vi "pH calibration.vi"(11 "pH index":i32) -> ()   [LabVIEW 2012]
uses:
  DAQ configuration/scale type.ctl
  DAQ configuration/Sensor buffer command.ctl
  global scale array.vi
panel:
  in  "Default Buffers":T1(array[cluster])=[{"Buffer"=4.0, "Calibrated"=FALSE, "V/T"=0.0013599919516459151}, {"Buffer"=7.0, "Calibrated"=FALSE, "V/T"=0.0}, {"Buffer"=10.0, "Calibrated"=FALSE, "V/T"=0.0}] {"V/T" format="%.2f"; "Buffer" format="%.2f"}
  out "name":string
  out "units":string
  in  "Temperature\nChannel":i32 min=0 step=1
  in  "Temperature":dbl[unit]=273.15 format="%.1f"
  in  "Temperature\ncompensated":bool
  out "XY Graph":cluster{dbl[], dbl[]}[](graph)
  in  "OK Button":bool
  in  "add buffer smooth interval (s)":sgl=1.0 format="%.3f"
  in  "Clear buffers":bool
  in  "Edit buffers":bool
  in  "Add buffer":bool
  out "Quit":bool
  out "Buffers":T1(array[cluster]) {"V/T" format="%.2f"; "Buffer" format="%.2f"}
  out "Sample Temperature":dbl[unit] format="%.2f"
  out "pH":dbl format="%.3f"
  out "pH voltage":sgl[unit] format="%.1f"
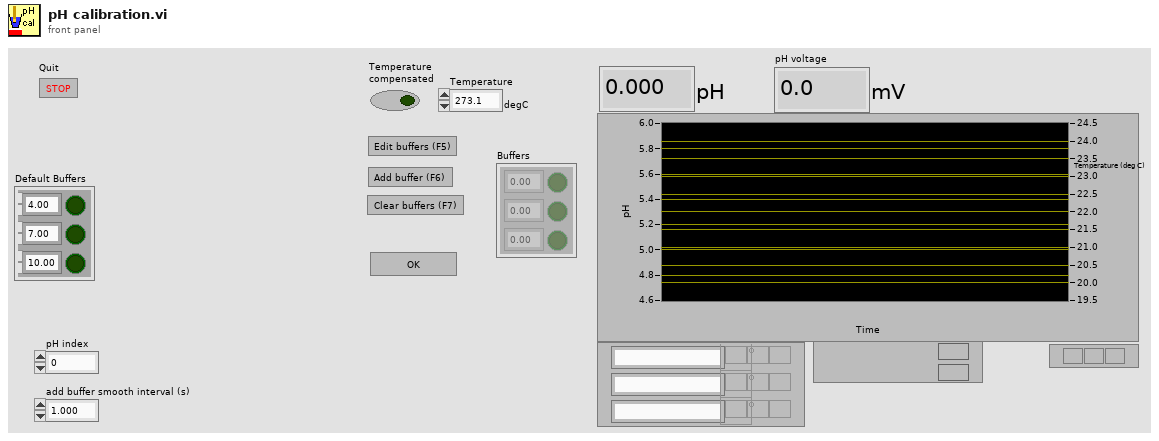
[diagram p1: front panel]
types:
  T1 = cluster{"Buffer":dbl, "Calibrated":bool, "V/T":dbl}[]
  T2 = typedef "scale type.ctl" = enum16{"Volts", "Polynomial", "Correspondence Table", "pH", "Dissolved Oxygen", "Quadratic"}
  T3 = typedef "Sensor buffer command.ctl" = enum16{"read average", "read recent", "read all", "write", "configure", "clear"}
  T4 = typedef "calib array.ctl" = T5[]
  T5 = typedef "conversion.ctl" = cluster{"conversion matrix":sgl[][], "units":string, "name":string, "scale type":T2, "offset (volts)":dbl, "second channel":i8, "correspondence table":T6, "offset (physical units)":dbl, "pH scale":T7, "D.O.":T8}
  T6 = typedef "correspondence table.ctl" = cluster{"physical units":dbl, "volts":dbl}[]
  T7 = typedef "pH scale.ctl" = cluster{"Buffers":cluster{"Buffer":dbl, "Calibrated":bool, "V/T":dbl}[], "Temperature":dbl}
  T8 = typedef "DO scale.ctl" = cluster{"Temperature":dbl, "K":dbl, "barometric pressure":dbl}
  T9 = cluster{"Buffer":dbl, "Calibrated":bool, "V/T":dbl}
  T10 = typedef "Sensor data.ctl" = cluster{" Sensor array":T11[], "Time":dbl}
  T11 = typedef "sensor cluster.ctl" = cluster{"voltage":sgl, "scaled":sgl, "units":string, "Out of Range":bool}
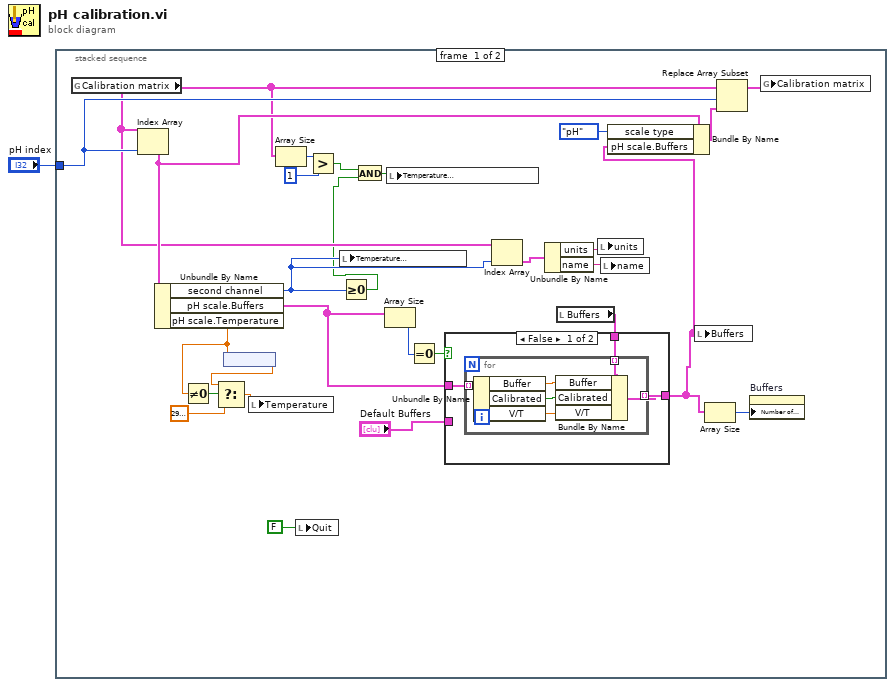
[diagram p0: block diagram]
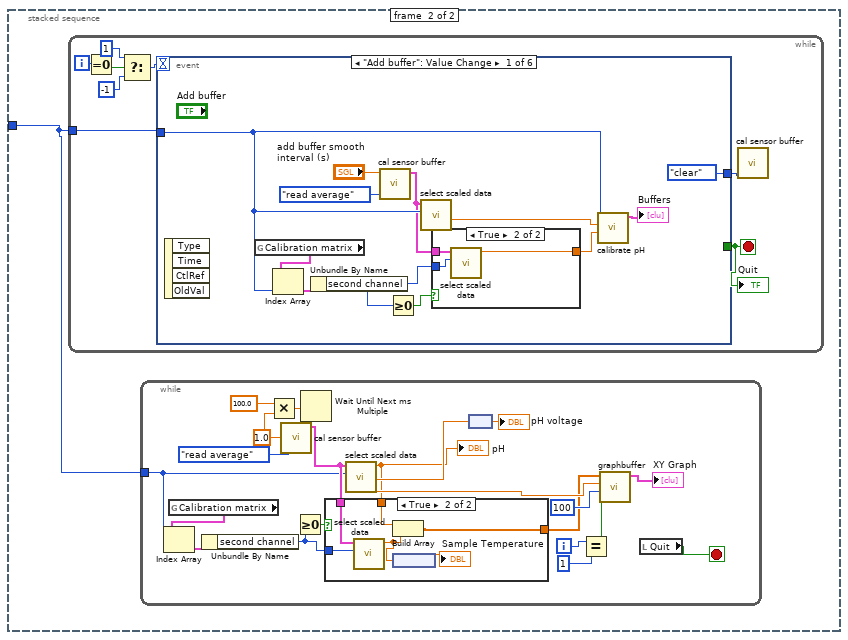
[diagram p3: hidden frame]
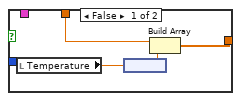
[diagram p4: hidden frame]
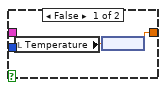
[diagram p5: hidden frame]
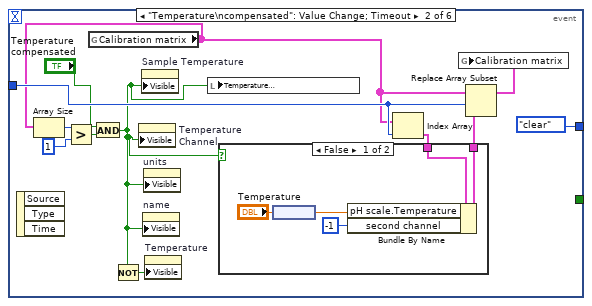
[diagram p6: hidden frame]
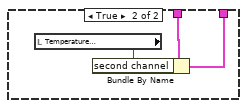
[diagram p7: hidden frame]
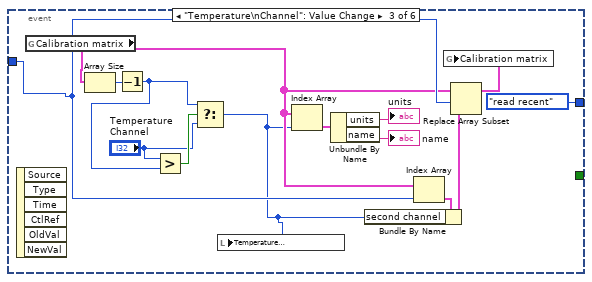
[diagram p8: hidden frame]
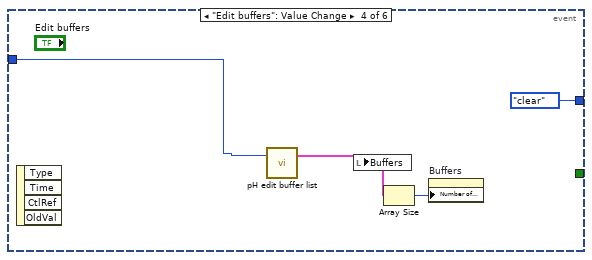
[diagram p9: hidden frame]
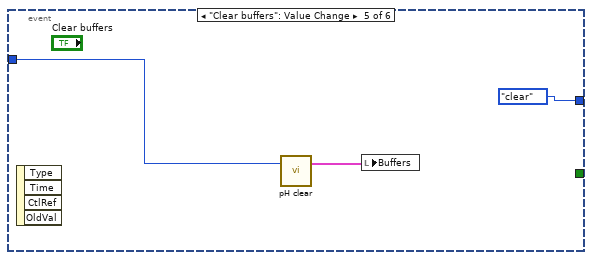
[diagram p10: hidden frame]
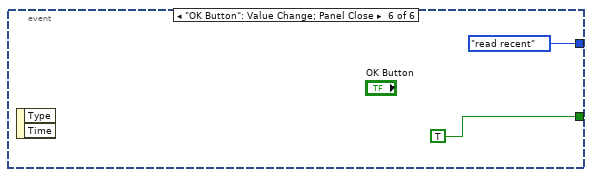
[diagram p11: hidden frame]
diagram:
  n1 = stacked-sequence {
    tunnel: "pH index" -> [w19 w40]
    frame #0 {
      n2 = global read "global scale array.vi" "Calibration matrix"() -> (w11:T4)
      n3 = Index Array(array=w11, index=w19) -> (element=w17:T5)
      n4 = Unbundle By Name(w17) -> ("second channel"=w27:i8, "pH scale.Buffers"=w23:T1, "pH scale.Temperature"=w7:dbl)
      n5 = Not Equal To 0?(x=w7) -> (x != 0?=w6:bool)
      n6 = node(w7) -> (w5:dbl[unit])
      n7 = Select(t=w5, s=w6, f=dbl[unit] 295.15) -> (s? t:f=w4:dbl[unit])
      n8 = local write "Temperature"(w4) -> ()
      n9 = Array Size(array=w11) -> (size(s)=w13:i32)
      n10 = local write "Quit"(FALSE ("Quit")) -> ()
      n11 = Greater?(x=w13, y=1) -> (0:w10:bool)
      n12 = local write "Temperature\nChannel"(w27) -> ()
      n13 = Greater Or Equal To 0?(x=w27) -> (x >= 0?=w9:bool)
      n14 = And(x=w10, y=w9) -> (x .and. y?=w8:bool)
      n15 = Array Size(array=w23) -> (size(s)=w21:i32)
      n16 = local write "Temperature\ncompensated"(w8) -> ()
      n17 = Equal To 0?(x=w21) -> (x = 0?=w22:bool)
      n18 = Index Array(array=w11, index=w27) -> (element=w26:T5)
      n19 = Unbundle By Name(w26) -> ("units"=w25:string, "name"=w24:string)
      n20 = local read "Buffers"() -> (w28:T1)
      n21 = case shown="False" w22 {
        tunnel: w23 -> [w32 _]
        tunnel: w28 -> [w31 _]
        tunnel: [w30 w39] -> w14
        tunnel: "Default Buffers" -> [_ w39]
        frame False {
          n22 = for {
            tunnel: w32 -> [w38] mode=indexing
            tunnel: w31 -> [w37] mode=indexing
            tunnel: [w34] -> w30 mode=indexing
            n23 = Unbundle By Name(w38) -> ("Buffer"=w36:dbl, "Calibrated"=w35:bool, "V/T"=w33:dbl)
            n24 = Bundle By Name(cluster=w37, "Buffer"=w36, "Calibrated"=w35, "V/T"=w33) -> (w34:T9)
          }
        }
        frame True {
        }
      }
      n25 = local write "units"(w25) -> ()
      n26 = local write "name"(w24) -> ()
      n27 = Bundle By Name(cluster=w17, "scale type"=scale_type."pH", "pH scale.Buffers"=w14) -> (w16:T5)
      n28 = local write "Buffers"(w14) -> ()
      n29 = Array Size(array=w14) -> (size(s)=w29:i32)
      n30 = Replace Array Subset(array=w11, new element=w16, index=w19) -> (w18:T4)
      n31 = property on="Buffers" class="Arr (strict)"("Number of Rows"=w29) -> ()  [unwired: 2 in, 2 out]
      n32 = global write "global scale array.vi" "Calibration matrix"(w18) -> ()
    }
    frame #1 {
      n33 = while {
        tunnel: w40 -> [w78]
        i -> [w74]
        stop <- w79 stop-if-true
        n34 = Equal To 0?(x=w74) -> (x = 0?=w73:bool)
        n35 = Select(t=1, s=w73, f=-1) -> (s? t:f=w75:i32)
        n36 = event shown="[0] \"Add buffer\": Value Change" {
          selector: _ -> [_ _ _ _ _ _]
          dyn-events: _ -> [_ _ _ _ _ _]
          timeout: w75 -> [_ _ _ _ _ _]
          tunnel: [_ _ _ _ _ TRUE ("OK Button")] -> w79
          tunnel: w78 -> [w91 w104 w126 w132 w136 _]
          tunnel: [Sensor_buffer_command."clear" ("command") Sensor_buffer_command."clear" ("command") Sensor_buffer_command."read recent" ("command") Sensor_buffer_command."clear" ("command") Sensor_buffer_command."clear" ("command") Sensor_buffer_command."read recent" ("command")] -> w72
          event "Add buffer": Value Change {
            n37 = event-data() -> ()  [unwired: 1 in, 4 out]
            n38 = global read "global scale array.vi" "Calibration matrix"() -> (w83:T4)
            n39 = Index Array(array=w83, index=w91) -> (element=w84:T5)
            n40 = Unbundle By Name(w84) -> ("second channel"=w82:i8)
            n41 = call "cal sensor buffer.vi"("command"=Sensor_buffer_command."read average", "smooth interval (s)"="add buffer smooth interval (s)") -> ("Sensor Data smoothed"=w88:T10)  [unwired: 3 in, 2 out]
            n42 = Greater Or Equal To 0?(x=w82) -> (x >= 0?=w81:bool)
            n43 = call "select scaled data.vi"("Sensor index"=w91, "Sensor Data"=w88) -> ("voltage"=w89:sgl)  [unwired: 4 in, 5 out]
            n44 = case shown="True" w81 {
              tunnel: w88 -> [_ w96]
              tunnel: [w92 w95] -> w86
              tunnel: w82 -> [_ w94]
              frame False {
                n45 = local read "Temperature"() -> (w93:dbl[unit])
                n46 = node(w93) -> (w92:dbl)
              }
              frame True {
                n47 = call "select scaled data.vi"("Sensor index"=w94, "Sensor Data"=w96) -> ("scaled"=w95:sgl)  [unwired: 4 in, 5 out]
              }
            }
            n48 = call "calibrate pH.vi"("index"=w91, "pH voltage"=w89, "Temperature"=w86) -> ("Buffers"=→"Buffers":T1)  [unwired: 7 in]
          }
          event "Temperature\ncompensated": Value Change; Timeout {
            n49 = event-data() -> ()  [unwired: 1 in, 3 out]
            n50 = global read "global scale array.vi" "Calibration matrix"() -> (w102:T4)
            n51 = Array Size(array=w102) -> (size(s)=w101:i32)
            n52 = Greater?(x=w101, y=1) -> (0:w99:bool)
            n53 = And(x="Temperature\ncompensated", y=w99) -> (x .and. y?=w97:bool)
            n54 = Not(x=w97) -> (.not. x?=w108:bool)
            n55 = property on="Temperature\nChannel" class="DigNum (strict)"("Visible"=w97) -> ()  [unwired: 2 in, 2 out]
            n56 = property on="Sample Temperature" class="DigNum (strict)"("Visible"=w97) -> ()  [unwired: 2 in, 2 out]
            n57 = property on="name" class="Str"("Visible"=w97) -> ()  [unwired: 2 in, 2 out]
            n58 = property on="units" class="Str"("Visible"=w97) -> ()  [unwired: 2 in, 2 out]
            n59 = property on="Temperature" class="DigNum (strict)"("Visible"=w108) -> ()  [unwired: 2 in, 2 out]
            n60 = local write "Temperature\ncompensated"(w97) -> ()
            n61 = Index Array(array=w102, index=w104) -> (element=w106:T5)
            n62 = case shown="False" w97 {
              tunnel: w106 -> [w113 w115]
              tunnel: [w112 w114] -> w105
              frame False {
                n63 = node("Temperature") -> (w110:dbl)
                n64 = Bundle By Name(cluster=w113, "pH scale.Temperature"=w110, "second channel"=i8 -1) -> (w112:T5)
              }
              frame True {
                n65 = local read "Temperature\nChannel"() -> (w116:i32)
                n66 = Bundle By Name(cluster=w115, "second channel"=w116) -> (w114:T5)
              }
            }
            n67 = Replace Array Subset(array=w102, new element=w105, index=w104) -> (w107:T4)
            n68 = global write "global scale array.vi" "Calibration matrix"(w107) -> ()
          }
          event "Temperature\nChannel": Value Change {
            n69 = event-data() -> ()  [unwired: 1 in, 6 out]
            n70 = global read "global scale array.vi" "Calibration matrix"() -> (w123:T4)
            n71 = Array Size(array=w123) -> (size(s)=w122:i32)
            n72 = Decrement(x=w122) -> (x-1=w120:i32)
            n73 = Greater?(x="Temperature\nChannel", y=w120) -> (0:w121:bool)
            n74 = Select(t=w120, s=w121, f="Temperature\nChannel") -> (s? t:f=w118:i32)
            n75 = local write "Temperature\nChannel"(w118) -> ()
            n76 = Index Array(array=w123, index=w118) -> (element=w130:T5)
            n77 = Unbundle By Name(w130) -> ("units"=→"units":string, "name"=→"name":string)
            n78 = Index Array(array=w123, index=w126) -> (element=w124:T5)
            n79 = Bundle By Name(cluster=w124, "second channel"=w118) -> (w125:T5)
            n80 = Replace Array Subset(array=w123, new element=w125, index=w126) -> (w127:T4)
            n81 = global write "global scale array.vi" "Calibration matrix"(w127) -> ()
          }
          event "Edit buffers": Value Change {
            n82 = event-data() -> ()  [unwired: 1 in, 4 out]
            n83 = call "pH edit buffer list.vi"("index"=w132) -> ("Buffers out"=w133:T1)  [unwired: 2 in]
            n84 = local write "Buffers"(w133) -> ()
            n85 = Array Size(array=w133) -> (size(s)=w134:i32)
            n86 = property on="Buffers" class="Arr (strict)"("Number of Rows"=w134) -> ()  [unwired: 2 in, 2 out]
          }
          event "Clear buffers": Value Change {
            n87 = event-data() -> ()  [unwired: 1 in, 4 out]
            n88 = call "pH clear.vi"("index"=w136) -> ("Buffers"=w137:T1)  [unwired: 2 in]
            n89 = local write "Buffers"(w137) -> ()
          }
          event "OK Button": Value Change; Panel Close {
            n90 = event-data() -> ()  [unwired: 1 in, 2 out]
          }
        }
        "Quit" <- w79
        n91 = call "cal sensor buffer.vi"("command"=w72) -> ()  [unwired: 4 in, 3 out]
      }
      n92 = while {
        tunnel: w40 -> [w48]
        i -> [w42]
        stop <- w61 stop-if-true
        w56 = sgl 1.0 ("smooth interval (s)")
        n93 = global read "global scale array.vi" "Calibration matrix"() -> (w50:T4)
        n94 = Index Array(array=w50, index=w48) -> (element=w49:T5)
        n95 = Unbundle By Name(w49) -> ("second channel"=w46:i8)
        n96 = Multiply(x=100.0 ("y"), y=w56) -> (x*y=w58:dbl)
        n97 = call "cal sensor buffer.vi"("command"=Sensor_buffer_command."read average", "smooth interval (s)"=w56) -> ("Sensor Data smoothed"=w59:T10)  [unwired: 3 in, 2 out]
        n98 = Greater Or Equal To 0?(x=w46) -> (x >= 0?=w45:bool)
        n99 = Wait Until Next ms Multiple(millisecond multiple=w58) -> ()  [unwired: 1 out]
        n100 = call "select scaled data.vi"("Sensor index"=w48, "Sensor Data"=w59) -> ("voltage"=w47:sgl, "scaled"=w44:sgl, "Time"=w55:dbl)  [unwired: 4 in, 3 out]
        "pH" <- w44
        n101 = case shown="True" w45 {
          tunnel: w59 -> [_ w71]
          tunnel: w46 -> [_ w70]
          tunnel: w44 -> [w65 w69]
          tunnel: [w64 w68] -> w43
          frame False {
            n102 = local read "Temperature"() -> (w63:dbl[unit])
            n103 = node(w63) -> (w62:dbl)
            n104 = Build Array(w65, w62) -> (w64:dbl[])
          }
          frame True {
            n105 = call "select scaled data.vi"("Sensor index"=w70, "Sensor Data"=w71) -> ("scaled"=w66:sgl)  [unwired: 4 in, 5 out]
            n106 = Build Array(w69, w66) -> (w68:sgl[])
            n107 = node(w66) -> (→"Sample Temperature":sgl[unit])
          }
        }
        n108 = node(w47) -> (→"pH voltage":sgl[unit])
        n109 = Equal?(x=w42, y=1) -> (x = y?=w53:bool)
        n110 = call "graphbuffer.vi"("Reset"=w53, "history length"=u16 100, "Time"=w55, "data"=w43) -> ("Multiplot graph data"=→"XY Graph":cluster{dbl[], dbl[]}[])  [unwired: 5 in, 2 out]
        n111 = local read "Quit"() -> (w61:bool)
      }
    }
  }
